vi "Imports.vi"(6 "error in":errorcluster, 9 "PythonConverter in":refnum<class "PythonBDConverter.lvclass">) -> (0 "error out":errorcluster, 3 "PythonConverter out":refnum<class "PythonBDConverter.lvclass">, 4 "imports":string)   [LabVIEW 2014, in "PythonBDConverter.lvclass"]
uses:
  PythonBDConverter.lvclass
  PythonBDConverter.lvclass/PythonBDConverter.ctl
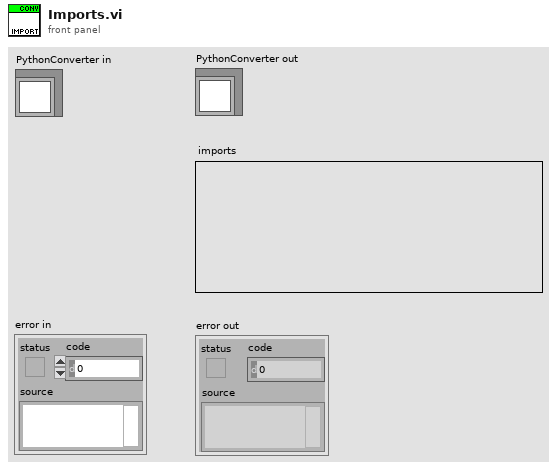
[diagram p1: front panel]
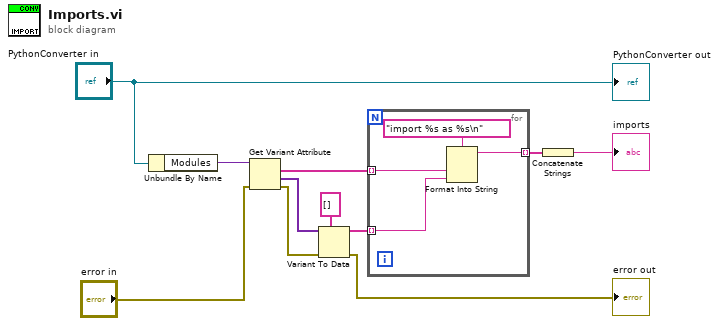
[diagram p0: block diagram]
diagram:
  n1 = Unbundle By Name("PythonConverter in") -> ("Modules"=w11:variant)
  n2 = Get Variant Attribute(Variant=w11, error in="error in") -> (names=w7:string[], values=w10:variant[], error out=w3:errorcluster)  [unwired: 2 in, 1 out]
  n3 = Variant To Data(error in=w3, type=string[] [], Variant=w10) -> (data=w8:string[], error out=→"error out":errorcluster)
  n4 = for {
    tunnel: w8 -> [w14] mode=indexing
    tunnel: w7 -> [w15] mode=indexing
    tunnel: [w12] -> w6 mode=indexing
    n5 = Format Into String(format string="import %s as %s\n", w15, w14) -> (resulting string=w12:string)  [unwired: 2 in, 1 out]
  }
  n6 = Concatenate Strings(w6) -> (→"imports":string)
  "PythonConverter out" <- "PythonConverter in"
